vi "Create DAQ Voltage Task.vi"(8 "error in (no error)":errorcluster, 9 "samples per channel":i32=100, 10 "physical channels":tag, 11 "Sampling Rate":dbl) -> (0 "error out":errorcluster, 3 "Refnum out":refnum<k21>)   [LabVIEW 2017]
uses:
  <vilib>/DAQmx/create/channels.llb/DAQmx Create Channel (AI-Voltage-Basic).vi
  <vilib>/DAQmx/configure/timing.llb/DAQmx Timing (Sample Clock).vi
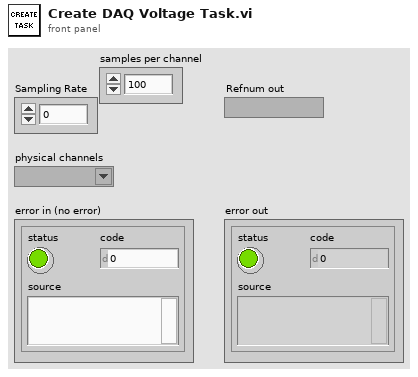
[diagram p1: front panel]
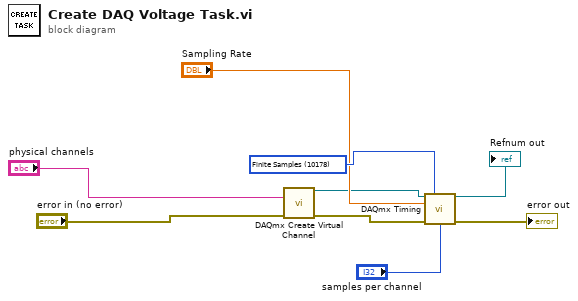
[diagram p0: block diagram]
diagram:
  w8 = 10178 items=["Finite Samples"=10178, "Continuous Samples"=10123, "Hardware Timed Single Point"=12522] ("sample mode")
  n1 = call-poly <vilib>:"DAQmx Create Virtual Channel.vi"("physical channels"="physical channels", "error in"="error in (no error)") -> ("task out"=w1:refnum<k21>, "error out"=w5:errorcluster)  [unwired: 12 in]
  n2 = call-poly <vilib>:"DAQmx Timing.vi"("task/channels in"=w1, "sample mode"=w8, "samples per channel"="samples per channel", "rate"="Sampling Rate", "error in"=w5) -> ("task out"=→"Refnum out":refnum<k21>, "error out"=→"error out":errorcluster)  [unwired: 9 in]
